vi "Orb_Calibration.vi"(0 "Voltage":dbl format="%.3f") -> (1 "Normalised Voltage":dbl format="%.3f", 2 "Orb Temp":dbl format="%.2f")   [LabVIEW 2010]
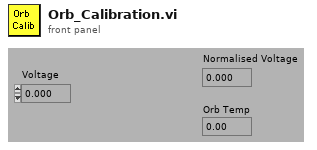
[diagram p1: front panel]
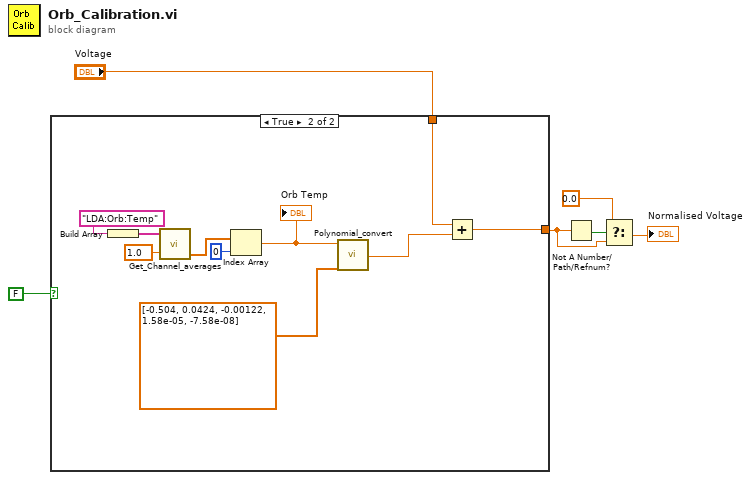
[diagram p0: block diagram]
diagram:
  n1 = case shown="True" FALSE ("Case Constant\n(See Context Help)") {
    tunnel: "Voltage" -> [w7 w11]
    tunnel: [w7 w9] -> w3
    frame False {
    }
    frame True {
      n2 = Build Array("LDA:Orb:Temp") -> (w16:string[])
      n3 = call "Get_Channel_averages.vi"("Desired Ch Names"=w16, "Averaging time (mins)"=1.0) -> ("number"=w14:dbl[])  [unwired: 1 in, 2 out]
      n4 = Index Array(array=w14, index=0 ("Index")) -> (element=w8:dbl)
      "Orb Temp" <- w8
      n5 = call "Polynomial_convert.vi"("Calib constants"=dbl[] [-0.504, 0.0424, -0.00122, 1.58e-05, -7.58e-08], "Voltage"=w8) -> ("Eng Values"=w10:dbl)  [unwired: 4 out]
      n6 = Add(x=w11, y=w10) -> (x+y=w9:dbl)
    }
  }
  n7 = Not A Number/Path/Refnum?(number/path/refnum=w3) -> (NaN/Path/Refnum?=w4:bool)
  n8 = Select(t=0.0, s=w4, f=w3) -> (s? t:f=→"Normalised Voltage":dbl)
